vi "Model Create.vi"(8 "error in (no error)":errorcluster) -> (0 "error out":errorcluster)   [LabVIEW 2015]
uses:
  Control Button/Exit.ctl
  Control Button/Save.ctl
  Control Button/Delete.ctl
  <vilib>/addons/database/Connection.llb/DB Tools Open Connec (String).vi
  Galobal variable_TI.vi
  <vilib>/addons/database/_DB Variant To Data/Database Variant To Data.xnode
  <vilib>/addons/database/NI_Database_API.lvlib
panel:
  out "error out 2":errorcluster
  out "new path":path
  out "Program seq. Name":string[](array[string])
  out "error out":errorcluster
  in  "Program Name":string
  in  "Edit Name":string
  in  "Program List":i32(listbox)
  in  "Delete":T1
  in  "Save":T2
  in  "Exit":T3
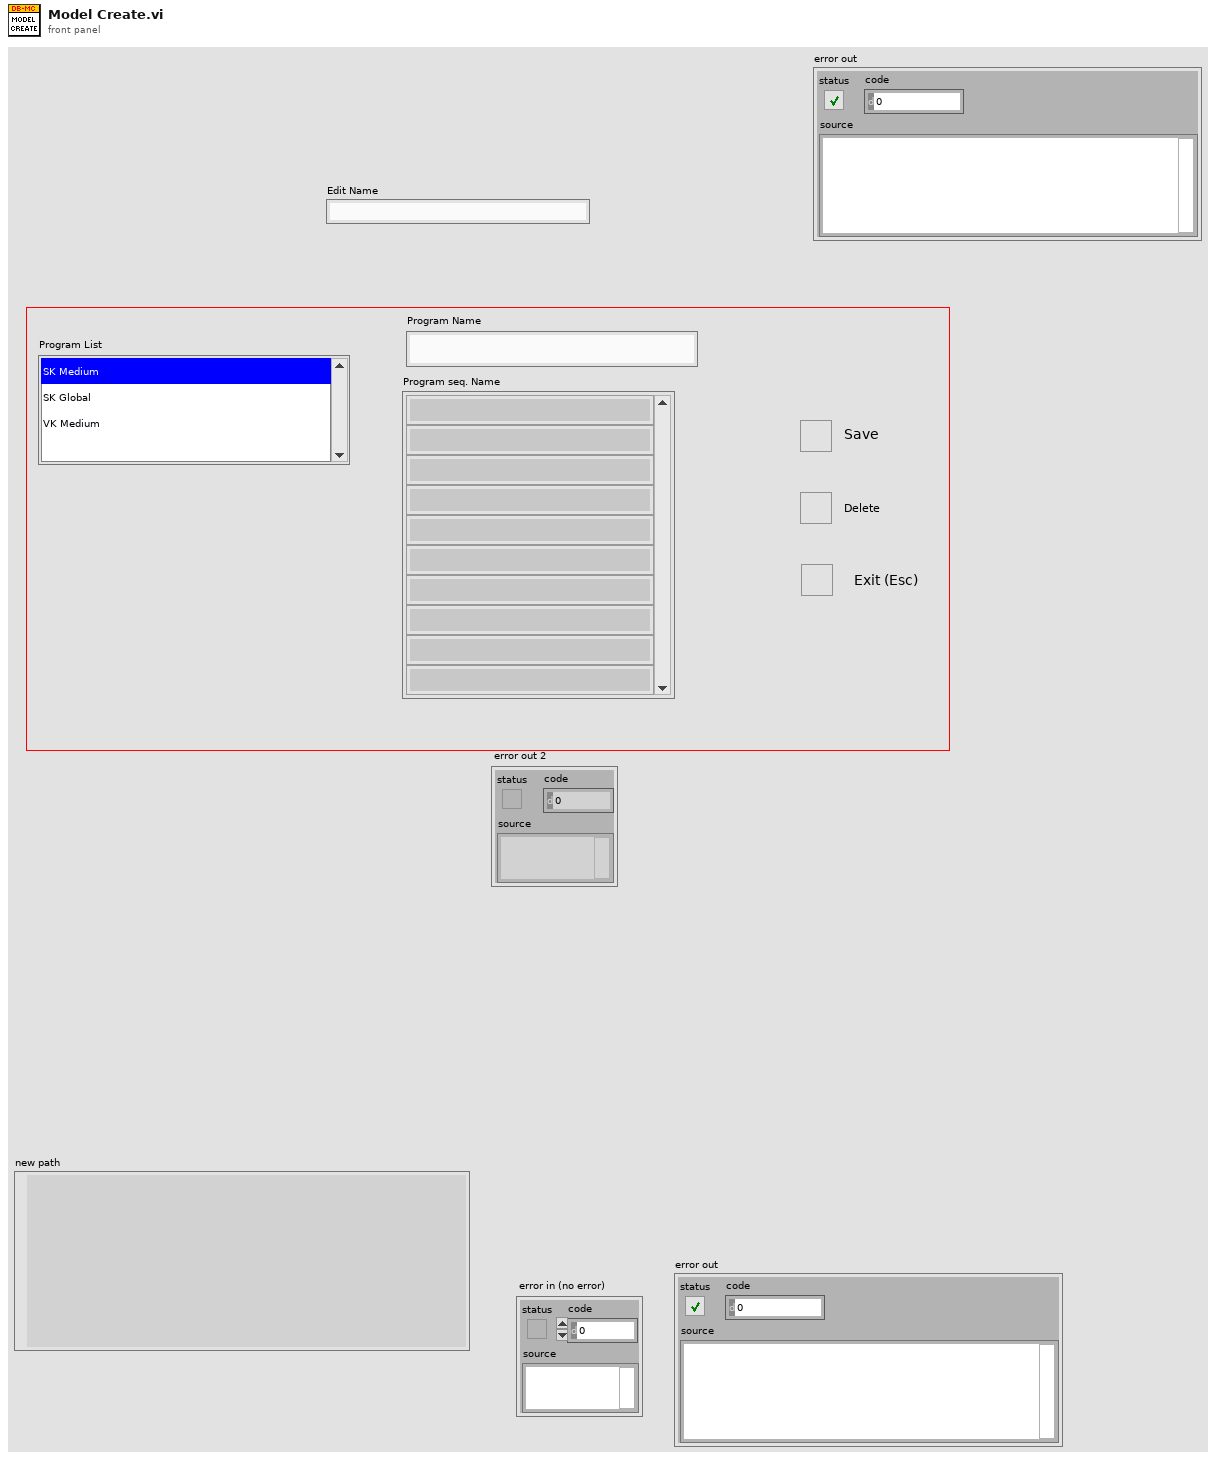
[diagram p1: front panel]
types:
  T1 = typedef "Delete.ctl" = bool
  T2 = typedef "Save.ctl" = bool
  T3 = typedef "Exit.ctl" = bool
  T4 = typedef "NI_Database_API.lvlib/Conn ObjectReference.ctl" = refnum<k1>
  T5 = enum16{"Left Button", "Center Button", "Right Button", "Window Close"}
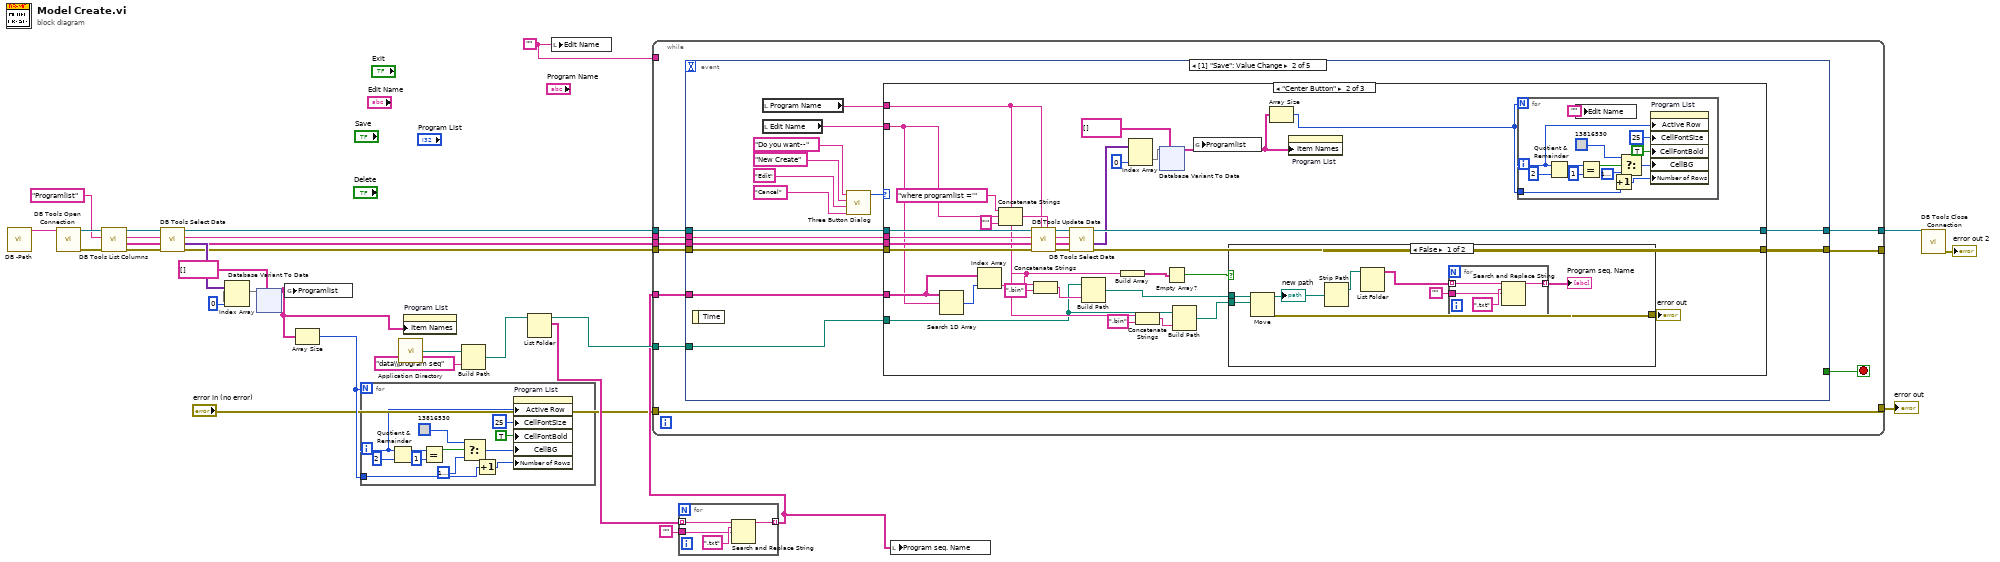
[diagram p0: block diagram]
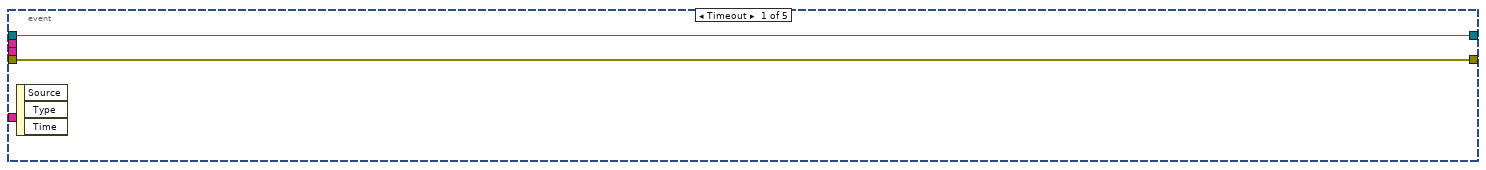
[diagram p2: hidden frame]
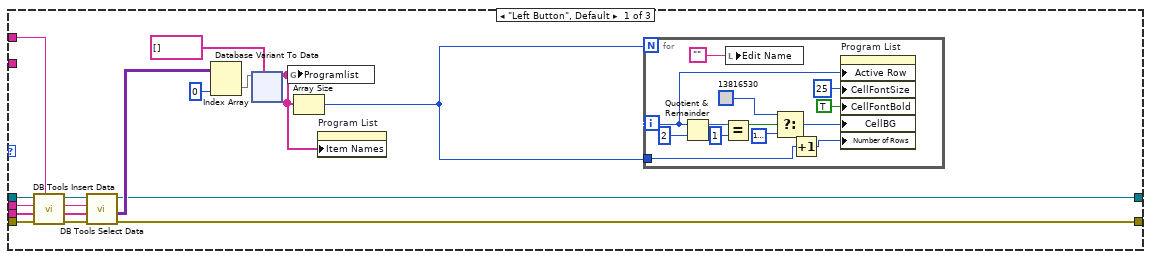
[diagram p3: hidden frame]
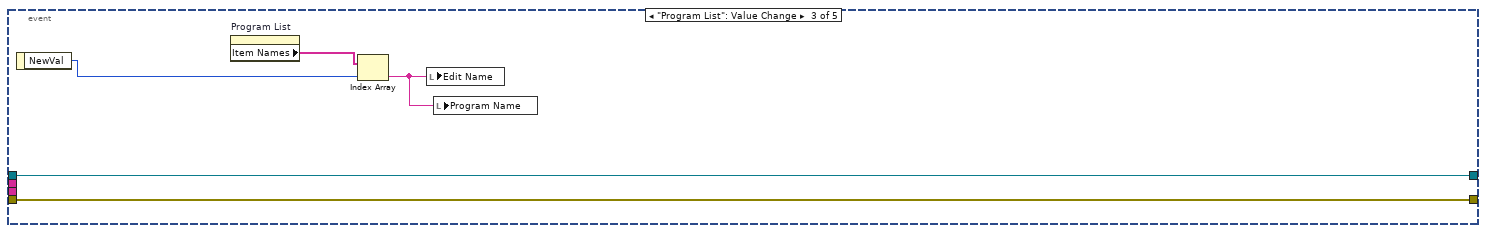
[diagram p6: hidden frame]
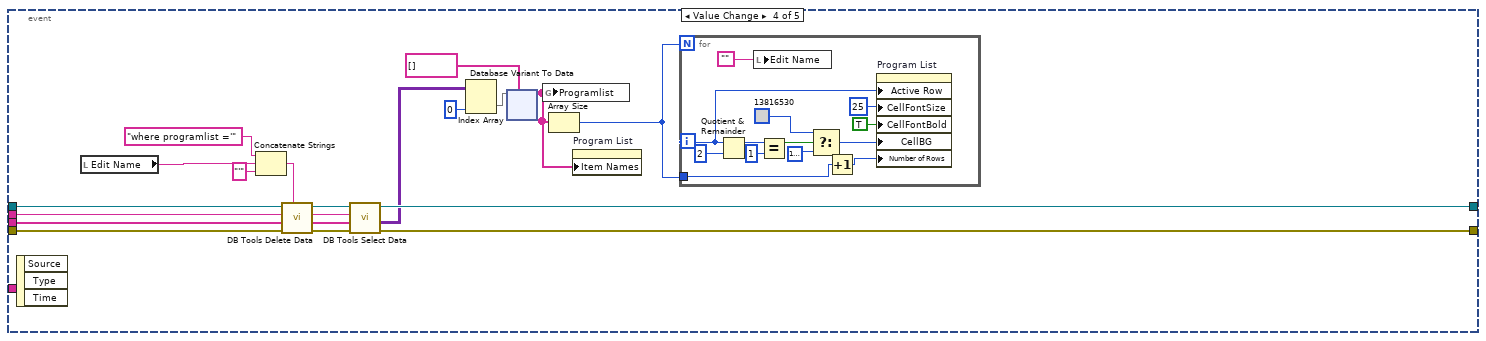
[diagram p7: hidden frame]
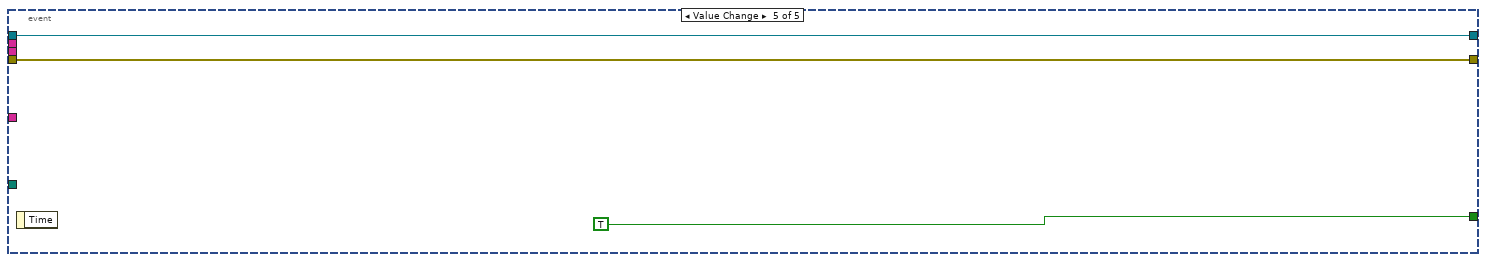
[diagram p8: hidden frame]
diagram:
  w10 = ""
  w13 = "Programlist" ("table")
  n1 = call "DB -Path.vi"() -> ("String"=w25:string)  [unwired: 11 in]
  n2 = call-poly <vilib>:"DB Tools Open Connection.vi"("connection information"=w25) -> ("error out"=w20:errorcluster, "connection reference"=w21:T4)  [unwired: 7 in]
  n3 = call <vilib>:"DB Tools List Columns.vi"("error in (no error)"=w20, "table"=w13, "connection reference"=w21) -> ("error out"=w18:errorcluster, "columns"=w14:string[], "connection reference out"=w19:T4)  [unwired: 1 in, 1 out]
  n4 = call <vilib>:"DB Tools Select Data.vi"("error in (no error)"=w18, "columns"=w14, "table"=w13, "connection reference"=w19) -> ("error out"=w15:errorcluster, "data"=w17:variant[][], "connection reference out"=w16:T4)  [unwired: 2 in]
  n5 = Index Array(array=w17, index (col)=0 ("disabled index (col)")) -> (element=w22:variant[])  [unwired: 1 in]
  n6 = xnode "Database Variant To Data"("database variant"=w22, "type"=string[] []) -> ("data"=w11:string[])  [unwired: 1 in, 1 out]
  n7 = global write "Galobal variable_TI.vi" "Programlist"(w11) -> ()
  n8 = Array Size(array=w11) -> (size(s)=w12:i32)
  n9 = for {
    N: w12 -> [_]
    tunnel: w12 -> [w29]
    i -> [w30]
    n10 = Quotient & Remainder(x=w30, y=2) -> (x-y*floor(x/y)=w38:i32)  [unwired: 1 out]
    n11 = Equal?(x=w38, y=1) -> (x = y?=w36:bool)
    n12 = Select(t=u32 13816530 ("Color Box"), s=w36, f=u32 16777225 ("Color Box")) -> (s? t:f=w33:u32)
    n13 = Increment(x=w29) -> (x+1=w28:i32)
    n14 = property on="Program List" class="LstBox (strict)"("Active Row"=w30, "CellFontSize"=u32 25 ("Active Row:Cell Font:Size"), "CellFontBold"=TRUE ("Active Row:Cell Font:Bold"), "CellBG"=w33, "Number of Rows"=w28) -> ()  [unwired: 2 in, 2 out]
  }
  n15 = call <vilib>:"Application Directory.vi"() -> ("Application Directory"=w27:path)
  n16 = property on="Program List" class="LstBox (strict)"("Item Names"=w11) -> ()  [unwired: 2 in, 2 out]
  n17 = Build Path(base path=w27, name or relative path="data\\program seq") -> (appended path=w9:path)
  n18 = List Folder(path=w9) -> (path out=w8:path, filenames=w7:string[])  [unwired: 3 in, 2 out]
  n19 = local write "Edit Name"(w10) -> ()
  n20 = for {
    tunnel: w7 -> [w43] mode=indexing
    tunnel: "" -> [w41]
    tunnel: [w40] -> w5 mode=indexing
    n21 = Search and Replace String(input string=w43, search string=".txt" ("replace string (\"\")"), replace string=w41) -> (result string=w40:string)  [unwired: 5 in, 3 out]
  }
  n22 = while {
    tunnel: w8 -> [w52]
    tunnel: w16 -> [w51]
    tunnel: w15 -> [w50]
    tunnel: w14 -> [w49]
    tunnel: w13 -> [w48]
    tunnel: [w47] -> w2
    tunnel: [w46] -> _
    tunnel: w10 -> [_]
    tunnel: w5 -> [w45]
    tunnel: [w44] -> w4
    tunnel: "error in (no error)" -> [w44]
    stop <- w53 stop-if-true
    n23 = event shown="[1] \"Save\": Value Change" {
      selector: _ -> [_ _ _ _ _]
      dyn-events: _ -> [_ _ _ _ _]
      timeout: _ -> [_ _ _ _ _]
      tunnel: [_ _ _ _ TRUE] -> w53
      tunnel: w52 -> [_ w57 _ _ _]
      tunnel: w51 -> [w55 w65 w238 w256 w309]
      tunnel: w50 -> [w54 w64 w237 w255 w308]
      tunnel: w49 -> [_ w62 _ w251 _]
      tunnel: w48 -> [_ w63 _ w252 _]
      tunnel: [w55 w61 w238 w250 w309] -> w47
      tunnel: [w54 w60 w237 w249 w308] -> w46
      tunnel: w45 -> [_ w58 _ _ _]
      event Timeout {
        n24 = event-data() -> ()  [unwired: 1 in, 3 out]
      }
      event Value Change {
        n25 = event-data() -> ()  [unwired: 1 in, 1 out]
        n26 = local read "Program Name"() -> (w56:string)
        n27 = local read "Edit Name"() -> (w59:string)
        n28 = call <vilib>:"Three Button Dialog.vi"("Right Button Text (\"Cancel\")"="Cancel" ("Right Button Text (\"Cancel\")"), "Center Button Text (\"No\")"="Edit" ("Center Button Text (\"No\")"), "Left Button Text (\"Yes\")"="New Create" ("Left Button Text (\"Yes\")"), "message"="Do you want--" ("Left Button Text (\"Yes\")")) -> ("Which Button?"=w70:T5)  [unwired: 7 in]
        n29 = case shown="\"Center Button\"" w70 {
          tunnel: w65 -> [w85 w168 w233]
          tunnel: w64 -> [w84 w167 w232]
          tunnel: w63 -> [w81 w161 _]
          tunnel: w62 -> [w80 w160 _]
          tunnel: [w74 w159 w233] -> w61
          tunnel: [w73 w158 w232] -> w60
          tunnel: w59 -> [_ w147 _]
          tunnel: w58 -> [_ w151 _]
          tunnel: w57 -> [_ w140 _]
          tunnel: w56 -> [w71 w141 _]
          frame "Left Button", Default {
            n30 = call <vilib>:"DB Tools Insert Data.vi"("data"=w71, "error in (no error)"=w84, "columns"=w80, "table"=w81, "connection reference"=w85) -> ("error out"=w82:errorcluster, "connection reference out"=w83:T4)  [unwired: 5 in]
            n31 = call <vilib>:"DB Tools Select Data.vi"("error in (no error)"=w82, "columns"=w80, "table"=w81, "connection reference"=w83) -> ("error out"=w73:errorcluster, "data"=w76:variant[][], "connection reference out"=w74:T4)  [unwired: 2 in]
            n32 = Index Array(array=w76, index (col)=0 ("disabled index (col)")) -> (element=w79:variant[])  [unwired: 1 in]
            n33 = xnode "Database Variant To Data"("database variant"=w79, "type"=string[] []) -> ("data"=w72:string[])  [unwired: 1 in, 1 out]
            n34 = global write "Galobal variable_TI.vi" "Programlist"(w72) -> ()
            n35 = Array Size(array=w72) -> (size(s)=w75:i32)
            n36 = property on="Program List" class="LstBox (strict)"("Item Names"=w72) -> ()  [unwired: 2 in, 2 out]
            n37 = for {
              N: w75 -> [_]
              tunnel: w75 -> [w88]
              i -> [w89]
              n38 = Quotient & Remainder(x=w89, y=2) -> (x-y*floor(x/y)=w97:i32)  [unwired: 1 out]
              n39 = Equal?(x=w97, y=1) -> (x = y?=w95:bool)
              n40 = local write "Edit Name"("") -> ()
              n41 = Select(t=u32 13816530 ("Color Box"), s=w95, f=u32 16777225 ("Color Box")) -> (s? t:f=w92:u32)
              n42 = Increment(x=w88) -> (x+1=w87:i32)
              n43 = property on="Program List" class="LstBox (strict)"("Active Row"=w89, "CellFontSize"=u32 25 ("Active Row:Cell Font:Size"), "CellFontBold"=TRUE ("Active Row:Cell Font:Bold"), "CellBG"=w92, "Number of Rows"=w87) -> ()  [unwired: 2 in, 2 out]
            }
          }
          frame "Center Button" {
            n44 = Search 1D Array(1D array=w151, element=w147) -> (index of element=w150:i32)  [unwired: 1 in]
            n45 = Index Array(array=w151, index=w150) -> (element=w146:string)
            n46 = Concatenate Strings("where programlist ='" ("condition"), w147, "'" ("string")) -> (w166:string)
            n47 = call <vilib>:"DB Tools Update Data.vi"("condition"=w166, "data"=w141, "error in (no error)"=w167, "columns"=w160, "table"=w161, "connection reference"=w168) -> ("error out"=w162:errorcluster, "connection reference out"=w163:T4)  [unwired: 4 in]
            n48 = Concatenate Strings(w146, ".bin" ("string")) -> (w144:string)
            n49 = call <vilib>:"DB Tools Select Data.vi"("error in (no error)"=w162, "columns"=w160, "table"=w161, "connection reference"=w163) -> ("error out"=w158:errorcluster, "data"=w152:variant[][], "connection reference out"=w159:T4)  [unwired: 2 in]
            n50 = Build Path(base path=w140, name or relative path=w144) -> (appended path=w143:path)
            n51 = Build Array(w146) -> (w149:string[])
            n52 = Index Array(array=w152, index (col)=0 ("disabled index (col)")) -> (element=w157:variant[])  [unwired: 1 in]
            n53 = Concatenate Strings(w141, ".bin" ("string")) -> (w139:string)
            n54 = xnode "Database Variant To Data"("database variant"=w157, "type"=string[] []) -> ("data"=w153:string[])  [unwired: 1 in, 1 out]
            n55 = Empty Array?(array=w149) -> (empty?=w148:bool)
            n56 = Build Path(base path=w140, name or relative path=w139) -> (appended path=w138:path)
            n57 = global write "Galobal variable_TI.vi" "Programlist"(w153) -> ()
            n58 = case shown="False" w148 {
              tunnel: w143 -> [w176 _]
              tunnel: w138 -> [w175 _]
              tunnel: [w174 _] -> w137
              frame False {
                n59 = Move(source path=w176, 10:w175) -> (error out=w174:errorcluster, 3:w173:path)  [unwired: 3 in, 1 out]
                "new path" <- w173
                n60 = Strip Path(path=w173) -> (stripped path=w172:path)  [unwired: 1 out]
                n61 = List Folder(path=w172) -> (filenames=w170:string[])  [unwired: 3 in, 3 out]
                n62 = for {
                  tunnel: w170 -> [w180] mode=indexing
                  tunnel: "" -> [w178]
                  tunnel: [w177] -> w169 mode=indexing
                  n63 = Search and Replace String(input string=w180, search string=".txt" ("replace string (\"\")"), replace string=w178) -> (result string=w177:string)  [unwired: 5 in, 3 out]
                }
                "Program seq. Name" <- w169
              }
              frame True {
              }
            }
            "error out" <- w137
            n64 = Array Size(array=w153) -> (size(s)=w154:i32)
            n65 = property on="Program List" class="LstBox (strict)"("Item Names"=w153) -> ()  [unwired: 2 in, 2 out]
            n66 = for {
              N: w154 -> [_]
              tunnel: w154 -> [w183]
              i -> [w184]
              n67 = Quotient & Remainder(x=w184, y=2) -> (x-y*floor(x/y)=w192:i32)  [unwired: 1 out]
              n68 = local write "Edit Name"("") -> ()
              n69 = Equal?(x=w192, y=1) -> (x = y?=w190:bool)
              n70 = Increment(x=w183) -> (x+1=w182:i32)
              n71 = Select(t=u32 13816530 ("Color Box"), s=w190, f=u32 16777225 ("Color Box")) -> (s? t:f=w187:u32)
              n72 = property on="Program List" class="LstBox (strict)"("Active Row"=w184, "CellFontSize"=u32 25 ("Active Row:Cell Font:Size"), "CellFontBold"=TRUE ("Active Row:Cell Font:Bold"), "CellBG"=w187, "Number of Rows"=w182) -> ()  [unwired: 2 in, 2 out]
            }
          }
          frame "Right Button" {
          }
        }
      }
      event "Program List": Value Change {
        n73 = event-data() -> ("NewVal"=w235:i32)  [unwired: 1 in]
        n74 = property on="Program List" class="LstBox (strict)"() -> ("Item Names"=w236:string[])  [unwired: 2 in, 2 out]
        n75 = Index Array(array=w236, index=w235) -> (element=w234:string)
        n76 = local write "Edit Name"(w234) -> ()
        n77 = local write "Program Name"(w234) -> ()
      }
      event Value Change {
        n78 = event-data() -> ()  [unwired: 1 in, 3 out]
        n79 = local read "Edit Name"() -> (w239:string)
        n80 = Concatenate Strings("where programlist ='" ("condition"), w239, "'" ("string")) -> (w240:string)
        n81 = call <vilib>:"DB Tools Delete Data.vi"("condition"=w240, "error in (no error)"=w255, "table"=w252, "connection reference"=w256) -> ("error out"=w253:errorcluster, "connection reference out"=w254:T4)  [unwired: 6 in]
        n82 = call <vilib>:"DB Tools Select Data.vi"("error in (no error)"=w253, "columns"=w251, "table"=w252, "connection reference"=w254) -> ("error out"=w249:errorcluster, "data"=w243:variant[][], "connection reference out"=w250:T4)  [unwired: 2 in]
        n83 = Index Array(array=w243, index (col)=0 ("disabled index (col)")) -> (element=w248:variant[])  [unwired: 1 in]
        n84 = xnode "Database Variant To Data"("database variant"=w248, "type"=string[] []) -> ("data"=w244:string[])  [unwired: 1 in, 1 out]
        n85 = global write "Galobal variable_TI.vi" "Programlist"(w244) -> ()
        n86 = Array Size(array=w244) -> (size(s)=w245:i32)
        n87 = property on="Program List" class="LstBox (strict)"("Item Names"=w244) -> ()  [unwired: 2 in, 2 out]
        n88 = for {
          N: w245 -> [_]
          tunnel: w245 -> [w259]
          i -> [w260]
          n89 = Quotient & Remainder(x=w260, y=2) -> (x-y*floor(x/y)=w268:i32)  [unwired: 1 out]
          n90 = local write "Edit Name"("") -> ()
          n91 = Equal?(x=w268, y=1) -> (x = y?=w266:bool)
          n92 = Select(t=u32 13816530 ("Color Box"), s=w266, f=u32 16777225 ("Color Box")) -> (s? t:f=w263:u32)
          n93 = Increment(x=w259) -> (x+1=w258:i32)
          n94 = property on="Program List" class="LstBox (strict)"("Active Row"=w260, "CellFontSize"=u32 25 ("Active Row:Cell Font:Size"), "CellFontBold"=TRUE ("Active Row:Cell Font:Bold"), "CellBG"=w263, "Number of Rows"=w258) -> ()  [unwired: 2 in, 2 out]
        }
      }
      event Value Change {
        n95 = event-data() -> ()  [unwired: 1 in, 1 out]
      }
    }
  }
  "error out" <- w4
  n96 = local write "Program seq. Name"(w5) -> ()
  n97 = call <vilib>:"DB Tools Close Connection.vi"("connection reference"=w2) -> ("error out"=→"error out 2":errorcluster)  [unwired: 6 in]
